vi "Thumbstick Value To Angle.vi"(0 "Vertical Axis":dbl, 1 "Horizontal Axis":dbl) -> (2 "Magnitude":dbl, 3 "Degrees":dbl, 4 "Radians":dbl)   [LabVIEW 2015, in "LabVIEW Interface for Arduino.lvlib"]
doc: "Convert thumbstick Horizontal Axis and Vertical Axis values to angle and magnitude."
uses:
  <vilib>/LabVIEW Interface for Arduino/LabVIEW Interface for Arduino.lvlib
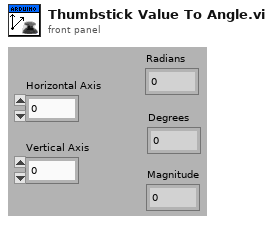
[diagram p1: front panel]
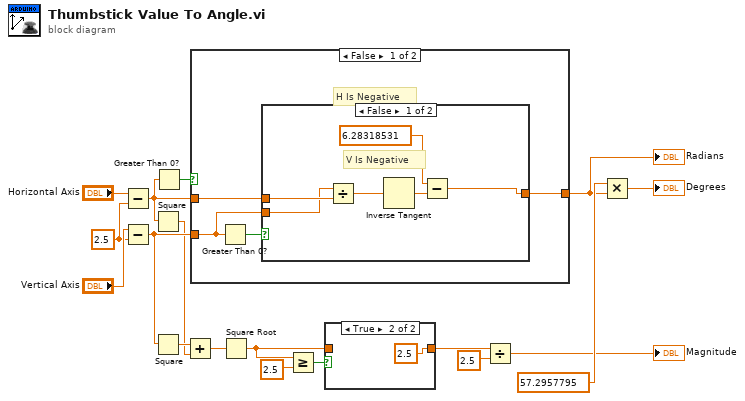
[diagram p0: block diagram]
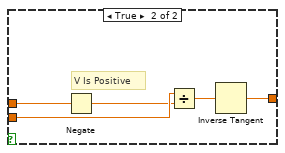
[diagram p3: hidden frame]
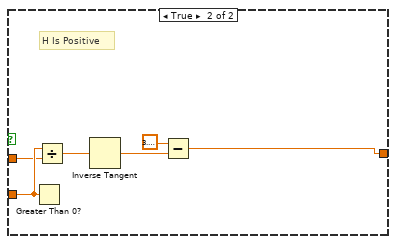
[diagram p4: hidden frame]
diagram:
  w15 = 2.5 ("y")
  n1 = Subtract(x="Horizontal Axis", y=w15) -> (x-y=w10:dbl)
  n2 = Subtract(x="Vertical Axis", y=w15) -> (x-y=w11:dbl)
  n3 = Square(x=w10) -> (x^2=w8:dbl)
  n4 = Square(x=w11) -> (x^2=w9:dbl)
  n5 = Greater Than 0?(x=w10) -> (x > 0?=w18:bool)
  n6 = Add(x=w9, y=w8) -> (x+y=w7:dbl)
  n7 = case shown="False" w18 {
    tunnel: w11 -> [w22 w39]
    tunnel: w10 -> [w21 w38]
    tunnel: [w20 w37] -> w13
    frame False {
      # "H Is Negative"
      n8 = Greater Than 0?(x=w22) -> (x > 0?=w19:bool)
      n9 = case shown="False" w19 {
        tunnel: w22 -> [w26 w33]
        tunnel: w21 -> [w27 w32]
        tunnel: [w25 w31] -> w20
        frame False {
          # "V Is Negative"
          n10 = Divide(x=w26, y=w27) -> (x/y=w28:dbl)
          n11 = Inverse Tangent(1:w28) -> (0:w24:dbl)
          n12 = Subtract(x=6.28318531, y=w24) -> (x-y=w25:dbl)
        }
        frame True {
          # "V Is Positive"
          n13 = Negate(x=w32) -> (-x=w30:dbl)
          n14 = Divide(x=w33, y=w30) -> (x/y=w29:dbl)
          n15 = Inverse Tangent(1:w29) -> (0:w31:dbl)
        }
      }
    }
    frame True {
      # "H Is Positive"
      n16 = Greater Than 0?(x=w39) -> ()  [unwired: 1 out]
      n17 = Divide(x=w39, y=w38) -> (x/y=w36:dbl)
      n18 = Inverse Tangent(1:w36) -> (0:w35:dbl)
      n19 = Subtract(x=3.141592653589793, y=w35) -> (x-y=w37:dbl)
    }
  }
  "Radians" <- w13
  n20 = Square Root(x=w7) -> (sqrt(x)=w4:dbl)
  n21 = Greater Or Equal?(x=w4, y=2.5) -> (x >= y?=w5:bool)
  n22 = case shown="True" w5 {
    tunnel: w4 -> [w40 _]
    tunnel: [w40 2.5] -> w3
    frame False {
    }
    frame True {
    }
  }
  n23 = Divide(x=w3, y=2.5) -> (x/y=→"Magnitude":dbl)
  n24 = Multiply(x=57.2957795, y=w13) -> (x*y=→"Degrees":dbl)
